vi "Draw Pixmap at Position.vi"(9 "Position":cluster{"left":i16, "top":i16}, 10 "Pixmap":T1, 11 "2D Picture In":picture) -> (3 "2D Picture":picture)   [LabVIEW 2022 SP3, in "FlexBlocks Support.lvlib"]
uses:
  FlexBlocks Support.lvlib
  <vilib>/picture/picture.llb/imagedata.ctl
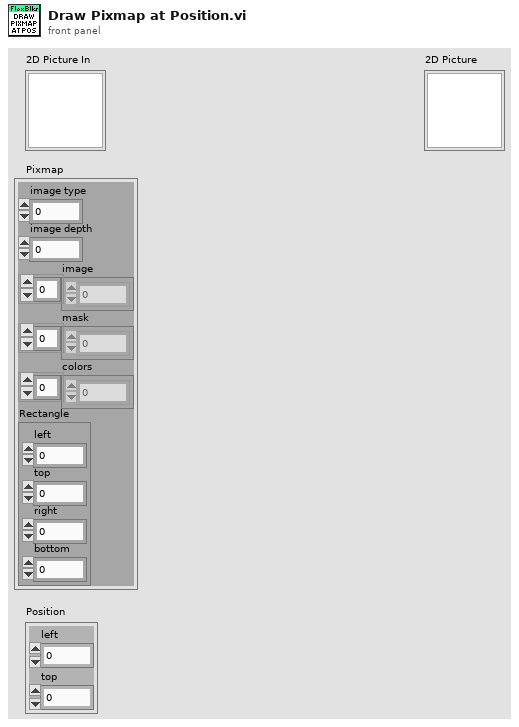
[diagram p1: front panel]
types:
  T1 = typedef "imagedata.ctl" = cluster{"image type":i32, "image depth":i32, "image":u8[], "mask":u8[], "colors":u32[], "Rectangle":cluster{"left":i16, "top":i16, "right":i16, "bottom":i16}}
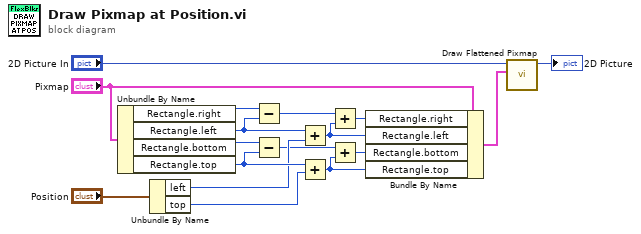
[diagram p0: block diagram]
diagram:
  n1 = Unbundle By Name("Pixmap") -> ("Rectangle.right"=w17:i16, "Rectangle.left"=w15:i16, "Rectangle.bottom"=w16:i16, "Rectangle.top"=w14:i16)
  n2 = Unbundle By Name("Position") -> ("left"=w12:i16, "top"=w11:i16)
  n3 = Subtract(x=w17, y=w15) -> (x-y=w10:i16)
  n4 = Subtract(x=w16, y=w14) -> (x-y=w9:i16)
  n5 = Add(x=w15, y=w12) -> (x+y=w6:i16)
  n6 = Add(x=w14, y=w11) -> (x+y=w4:i16)
  n7 = Add(x=w10, y=w6) -> (x+y=w7:i16)
  n8 = Add(x=w9, y=w4) -> (x+y=w5:i16)
  n9 = Bundle By Name(cluster="Pixmap", "Rectangle.right"=w7, "Rectangle.left"=w6, "Rectangle.bottom"=w5, "Rectangle.top"=w4) -> (w2:T1)
  n10 = call <vilib>:"Draw Flattened Pixmap.vi"("image data"=w2, "picture"="2D Picture In") -> ("new picture"=→"2D Picture":picture)  [unwired: 7 in]
